vi "Init control.vi"(7 "ctl in":refnum<class "ctl.lvclass">, 8 "error in":errorcluster) -> (0 "error out":errorcluster, 3 "ctl out":refnum<class "ctl.lvclass">)   [LabVIEW 2012, in "ctl.lvclass"]
uses:
  ctl.lvclass
  Control Class/_ResourceManager_v86/ResManager/ID_Resource info.ctl
  ctl.lvclass/ctl.ctl
  Control Class/_ResourceManager_v86/ResManager/IDCloneResMgr.lvlib
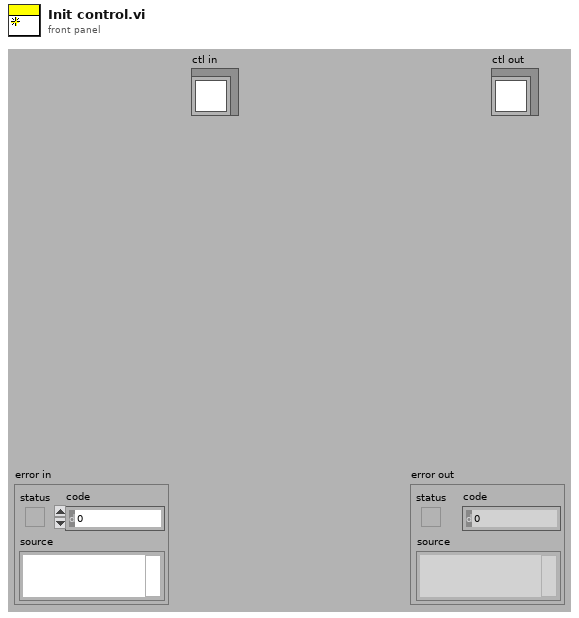
[diagram p1: front panel]
types:
  T1 = typedef "IDCloneResMgr.lvlib/ID_Resource info.ctl" = cluster{"type":u32, "id":i32, "name":string, "binary data":string}
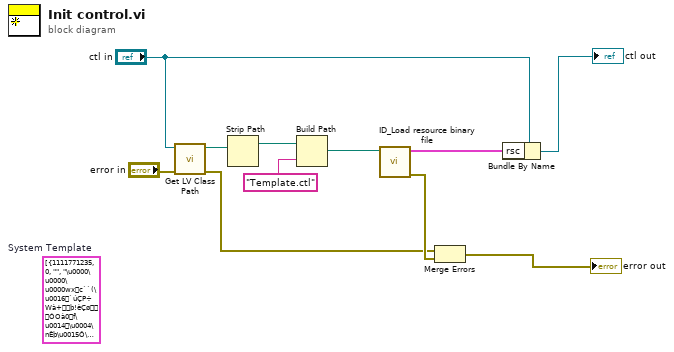
[diagram p0: block diagram]
diagram:
  (unwired) T1[] [{"type"=1111771235, "id"=0, "name"="", "binary data"="\u0000\u0000\u0000wxc``(\u0016`úÇP÷Wà+þ!èÇøÓOà0f\u0014\u0004\nÊþ\u0015Ô\u0006\u000bj³èª²1ªX1sHr\u001c\u0016ä\u0000q´h0üÿÿ_¥ã+Ë5\u0016\u001fYò\u001c\u0012\f\fÌ\f¸\f\u0000\u0004{\u0017´"}, {"type"=1111774021, "id"=0, "name"="", "binary data"="\u0000\u0000\u0000\u0007\u0000\u0000\u0001z"}, {"type"=1129270864, "id"=0, "name"="", "binary data"="\u0000\u0001"}, {"type"=1129333554, "id"=0, "name"="", "binary data"="\u0000\u0001"}, {"type"=1145455699, "id"=0, "name"="", "binary data"="\u0000\u0000\u0001\u0015xc`À\t\u0018\u0019\u0018X847Là?\u0010@Ä\u0005·Vò\u0001Ô\u000e\f6>1l@\u0000B1\u0002\u00153}\u00002\u0019À\u000e\u0007a¦?@ü\u000fY1#f\u0000Õ\u0001\u0014\u0018"}, {"type"=1146374224, "id"=0, "name"="", "binary data"="\u0000\u0002\u0000\u0010"}, {"type"=1179666531, "id"=0, "name"="", "binary data"="\u0000\u0000\u0004\u0006xS¿oÓ@\u0014~wuÜsià\\¨ \u0014ëÜ\u0004D°!è\u001a\u0017TT\n¨ø± \u00061T\u0004\u0012b\u0002©òâ¡,lþ\r\f\u0019X\u0011Ä\nY\u0015bghUK(6ïì\u0018÷G\u0010gÙïî½ï½ïî{g\u0000ò\u001c\rà¥ÏwÑ,õW{\u0004@©ð:ù\räTôYoÑ\u001402Ë.Ø.üÂè6FUÇ1ôOé7ÇÅûp3\u0018Ü \u0001½'{lÃic1pÊò«WH\u0000Ä>«(y»Ñj:Bzµ\nËGu4ßîe\n¯eäSZ\u0007°N\u0019:Î!älDxé?ÀgÂ;\u001f\u0001Ç\u0012 ]\fÞÈ­Iä!¼è!\u001c±/Rlÿêà\u0018Ft\fc}â\u000boåÙöê7½ã|\u0000\u0002Dy¨/KÕ\"ÀDßF%­ËÀWpu\u000bUR#]¥rT9r=RnÒv9¤'Ù\u0019.­tÍÑùv{­ÙhÅòq+&Ä82qÎ¡s\u001c·eýÕ5ë#³ö\\x\u0006²\b÷ÄA¹ÌPÀ\u001e®©Ö\u001a­GÍµó¨1O·Z\u0018@D[CSw÷ÈYiÔµ0\f\u0007Èc\u0012i\bo2¾jqL/Æ\u0017.N\u0019Ðxª¤ÓáÞÌ\u0001¯VÜß?ë>X\u000fÀöÇ¯ÈNb¯ØU\u001a\u00116nE[Þ'\u0013Ûâ\u000bóªo×&>f²Va/&z\u001dÅÄìE¶À7ñ7!>Ûd»ÊWeÉùB~Ðx[d9`xQª\u0000ä1½\t4òè0\r@çH\u001dt|q-çt\u000eýº\fËyø9tÉkÚép\u000f\nÃ*ë Û¢\"¦\n§á\u001aÚ\u00120\u0005ÇÁ\u0000#ü\u000e'1z\u0006ÖÃ\u0011Ç\f>MØÓñî\u000f&ñû\u000b"}, {"type"=1179669317, "id"=0, "name"="", "binary data"="\u0000\u0000\u0000\u0017\u0000\u0000\u0005N"}, {"type"=1179926850, "id"=128, "name"="", "binary data"="\u0000\u0001\u0000\u0002\u0000\u0003\u0000\u0005\u0000\u0000\u0000X\u0000\u000f\u0004\u0000\u0000\u0000\u0000\u000f\u0000Ø\u0000Õ\u0000\u0000\u0000a\u0000\u000f\u0004\u0000\u0000\u0000\u0000\u000f\u0000Ø\u0000Õ\u0000\u0000\u0000j\u0000\u000f\u0004\u0000\u0000\u0000\u0000\u000f\u0000Ø\u0000Õ\u0000\u0000\u0000s€\u0000„\u0000€\u0000\u0000\u000f\u0000Ø\u0000Õ\u0000\u0000\u0000u€\u0000„\u0000€\u0000\u0000\u000f\u0000Ø\u0000Õ\bSegoe UI\bSegoe UI\bSegoe UI\u00011\u00012"}, {"type"=1212765012, "id"=0, "name"="", "binary data"="\u0000\u0000\u0000\u0002\u0000\u0000\u0004\u0000\u0000\u0000\u0000\u000b\u0000\u0000\u0000\u0000\u0000\u0000\u0000\u0000\u0000\u0000\u0000\u0000\u0000\u0000\u0000\u0000\u0000\u0000\u0000\u0000\u0000\u0000\u0000\u0000\u0000\u0000\u0000\u0000"}, {"type"=1229147982, "id"=0, "name"="", "binary data"="ÿÿÿÿ\u0000\u0000\u0001\u0000\u0000\u0001@\u0000\u0001à\u0000\u0001ð\u0000\u0001\u0000\u0000\u0001à\u0000\u0001à\u0000\u0001à\u0000\u0001à\u0000\u0001ä\u0000\u0001ì\u0000\u0001Ô\u0000\u0001¤\u0000\u0001Ô\u0000\u0001ì\u0000\u0001ä\u0000\u0001à\u0000\u0001à0\u0001à,\u0001àã\u0001à$Áà.9à$Á\u0000ã\u0001ð,\u0001à0\u0001@\u0000\u0001\u0000\u0000\u0001\u0000\u0000\u0001ÿÿÿÿ"}, {"type"=1279877732, "id"=0, "name"="", "binary data"="\u0000\u0001BDHP\fTemplate.ctl\u0000\u0000\u0000\u0000\u0000\u0000\u0000\u0000\u0003"}, {"type"=1279878259, "id"=0, "name"="", "binary data"="\u0000\u0001VIDS\fTemplate.ctl\u0000\u0000\u0000\u0000\u0000\u0000\u0000\u0000\u0003"}, {"type"=1279878768, "id"=0, "name"="", "binary data"="\u0000\u0001FPHP\fTemplate.ctl\u0000\u0000\u0000\u0000\u0000\u0000\u0000\u0000\u0003"}, {"type"=1279882857, "id"=0, "name"="", "binary data"="\u0000\u0001LVCC\fTemplate.ctl\u0000\u0000\u0000\u0000\u0000\u0000\u0000\u0000\u0003"}, {"type"=1280725842, "id"=0, "name"="Template.ctl", "binary data"="\b`\u0001\u0000\u0000\u0000\u0000 \u0000\u0000\u0000\u0000\u0000\u0000\u0004\u0000\u0003\u0000<\u0000¼\u0000\u001f@\u0002\u0000\u0000\u0000\u0000\u0001\u0000\u0001\u0000\u0006ÿÿÿÿ\u0000\u0000\u0000\u0000\u0000\u0000\u0000\u0000\u0000\u0000\u0000\u0000m»+ånfN´ª¬¬\u001bcóz\u0000\u0000\u0000\f\u0000\u0000\u0000\u0010\u0000\u0000\u0000\u0002ñrÈFô}vG§qnâÃ¸Ô\u001dÙ\u0000²\u0004é\tìøB~\u0000\u0000@\u0000\u0000\u0000\u0000\u0000"}, {"type"=1296975689, "id"=2, "name"="", "binary data"="PNG\r\n\u001a\n\u0000\u0000\u0000\rIHDR\u0000\u0000\u0000\u0016\u0000\u0000\u0000\u0016\b\u0006\u0000\u0000\u0000Ä´l;\u0000\u0000\u0000\u0004gAMA\u0000\u0000¯È7\u0005é\u0000\u0000\u0000\u0019tEXtSoftware\u0000Adobe ImageReadyqÉe<\u0000\u0000\u0004:IDATxÚbüÿÿ?\u0003-\u0000@\u000011Ð\b\u0000\u0004 pÜ\u0000\u0004(¸|N\f´\u00023Û±\b±\u0010t\u0019àÀ#y»Á\u0006/ÎÙù<v!\u0015i1Ñ\u00154V4\u00144ª+ ÊHæL7úÊ°\u0006¯×²¥×{÷å;¿\u0000¢ØÅà üó·EJLt]¨µ¨\u0010<H\u001c X(1ôÏ\fl\fëLuÔÌãÍõ\u00197]½ÇðêÉÇÍ 9\u0000\"ËÅ@üûÏ_\u0006\u000eÖóA6\u0006\u0016]nögî¿dØuäæ¥¿ÿÔ\u0000\u0004\u0010\u000bÔ;\u0002ÿÿýg\u00032_\u0011ôú¿ÿ\fß~ýí\u0013\u0015ÈIrÐd\rWVbXxõ.ÃâÝ×\u001e3þftcd\u0005E\u0004\u0003\u0003@\u0000\ræàd?öAôÏû¿^Ì\f\f§q\u0019ú÷ïÉ_,ÿ×iéHXä;ê08\b\u000b3Ì¹yaúæ«\u001f\u0018¿ýscæfxùñ\u001fX-@\u0000[ÅÖZNmÛß?ÿÁ~E\u0003¿ÿ\u000b`âe>ïf§hÑìiÍ`%,É°êÁcÙ[îü`üÀ\u0018ÉÆÌvå/\u001b\u0003Ëo\u000e°z\u0000\u0002\u001büþé3\n\\Ü\fÁnª\"Xÿ\u001føûç¿,Âë\f\f¿þüÉ+Ã¶:ÅOW¼ÜÖASaë£G\fÓ×Ýÿûëù¿$nv¶\u001dìÿ¸\u0019¸~\n0ð|\u0011\u0001ë\u0003\b °Áÿ¿2M>qæýÿ0\u001d\u000b\u0006\u001fG5\u001f÷üûÃÀ\u0001²à'óß\u0013*\u0006..."}, {"type"=1296975689, "id"=3, "name"="", "binary data"="PNG\r\n\u001a\n\u0000\u0000\u0000\rIHDR\u0000\u0000\u0000\u0000\u0000\u0000\u001e\b\u0006\u0000\u0000\u0000à§ÆÅ\u0000\u0000\u0000\u0001sRGB\u0000®Î\u001cé\u0000\u0000\u0000\u0004gAMA\u0000\u0000±\u000büa\u0005\u0000\u0000\u0000\tpHYs\u0000\u0000\u000eÃ\u0000\u0000\u000eÃ\u0001Ço¨d\u0000\u0000\u0000\u0019tEXtSoftware\u0000Paint.NET v3.5.1Nç8ù\u0000\u0000\u0001LIDAThCíA.DA\u0014EÿÈ\u0012\fÌíÂ\u0016L{#¬Â\u001aÌåK\u0004ÐBBÆ\u001f MH´DcÐ§êu{I%vpO%7\\§Î»õ'Õ4óµÜÛ´fe\b1X\\Ýxÿ;ÿÙ7o~ïìÎXZ\u0004.»ç2ø[y×ÛMnµ¶«EÝ\u0006¶?4¿\rJ\u001b¤(bÿ\u0012 ö\u0010 h\u0003ü×þÑ\b?ÓdDAð9IöõMT\u0019T\"\u0014\u0019&\u0003D@~\u001f~D@ZñÇÔ.h\u0004$Ð =\"Ð~\u0013\b/¯\u0013#º\f\u0010\u0001ð\u0002\b\u0011\u001eÆFt\u0019 \u0002\u0003à\u0005\bPpß½\u0019Ñe\u0010\u0004º\u0012³G\u0004Ðo\u0010áúfdD\u0001\"0\u0000^\u0000\bW\u0011=\u0006\b\u0017çFt\u0019D#tFt\u0019¸\bùÙµGÇvx0 ¢\f\u0003ñämgw\u001f\u0011\u0004E]\u000bó\u001f9,ð\bVï\u0001pi¼\u0006¿ÊÊÚí¥Ö\u0000\u0000\u0000\u0000IEND®B`"}, {"type"=1296975689, "id"=4, "name"="", "binary data"="PNG\r\n\u001a\n\u0000\u0000\u0000\rIHDR\u0000\u0000\u0000\u0000\u0000\u0000\u001e\b\u0006\u0000\u0000\u0000à§ÆÅ\u0000\u0000\u0000\u0001sRGB\u0000®Î\u001cé\u0000\u0000\u0000\u0004gAMA\u0000\u0000±\u000büa\u0005\u0000\u0000\u0000\tpHYs\u0000\u0000\u000eÃ\u0000\u0000\u000eÃ\u0001Ço¨d\u0000\u0000\u0000\u0019tEXtSoftware\u0000Paint.NET v3.5.1Nç8ù\u0000\u0000\u0001yIDAThCí1N\u0002Q\u0010W\u000fá\r¸\u0017°°õ\u001c\u0016ÔVÀÞR\u0003\r\u0018³\u0016lÄd7D\b\u00180Á\u0004*M°m\u0004Â\u000eoî-µäÿ7ùYÚ÷Í7ó( øyJG§\u0012ì\u0019 \u0006{'i^ÿ>8>óðÁ\"P\u000fCÑÚ{\tÜ$\u0018Tªu©U#\u0006Áåu$Îç@¯«FÂ\u00003ð?\tôã&ì0À\fLfÔ\u0013\u0006pÛê\tË\"°\u0001ü\u00000\u0011âd(\f.\u0003°\rÐûnj°\"üg²\b÷Ý0¸\f(\u0002\u001bÀ\u000f\u0000@\u0011\"<\f&Âà2°@\tp%ÐÚ\b£§\u0017ap\u0019P\u00046\u001f\u0000\u0014\"\u0014E\u0018O¦Âà2°@\tp%ÐÚS\u0004NB\u0013\bÓ×T\u0018\\\u0006&ÂÛl.yféB\u0018,\u0006&Âûb%yæËµ08\fô\u000fü&\u0016~ùéòµ\u0015Ä  Be\u0007kÅ§5\u0011ÜÚ46\u0012ûÃïm'wþ\u001dýÒ¸ë¢À=vçqü»ò¦ko\u000eÅ.`ñ\u0016õ6ÐA \u000el\u0000>¸¬pýùàÕ\u0000\u0000\u0000\u0000IEND®B`"}, {"type"=1296975689, "id"=5, "name"="", "binary data"="PNG\r\n\u001a\n\u0000\u0000\u0000\rIHDR\u0000\u0000\u0000\u0000\u0000\u0000\u001e\b\u0006\u0000\u0000\u0000à§ÆÅ\u0000\u0000\u0000\u0001sRGB\u0000®Î\u001cé\u0000\u0000\u0000\u0004gAMA\u0000\u0000±\u000büa\u0005\u0000\u0000\u0000\tpHYs\u0000\u0000\u000eÃ\u0000\u0000\u000eÃ\u0001Ço¨d\u0000\u0000\u0000\u0019tEXtSoftware\u0000Paint.NET v3.5.1Nç8ù\u0000\u0000\u0002$IDAThCí=KÃ`\u0014ó+ü\u0007Îº¸¨.ÚAÐEtÓÁAA¤ÅA+\bÚ*(K¥  ¢KµT\n\u0015EAé`±â÷'Tñ£\u0015¬&iâõ½\tM\u0002NÃ½CÚ¥s{îKá$ñ\u001a\b-\u0007Ê[ Õö³\byPÖ4\f¡\u0015@\u0006\u0010ÞéEÈ>¥\u0001r)\u0016!\u000fä·cÀì\r\u0018°\tÞ¯×@K\u000f~>Á\"ä\u0001fÙ\u001bÛ\u0000×ÁÏÝ\t®³\by`d~?o\u001e\u0007\f\u0010nf\u0019\u0004B\u0000\u0014\u0007\u001eAÀì-\u0010ô«\u0019\u0006(\b½\rØ¼\u001aè­Åâ¹Ð\u0006ádA Ú\b'#v#hi¿\u0000Á\u000f²¦³\by \u001dù\u0019\u0004êà3\b¦¾\u0014ìn\u0010\u000e½ \t}}ë,B\u001e\u0014R>»Ï±\u001a\u0018\u0004\u0003À \u0010úR-ï\u0006!Ù\rd\u000f|æu\u0016!\u000f0sMdoý\u001f\u0018\u0004zCà\u0002¡°ß\t\u000eÈ}h,B\u001e¨»Õ\b\f\u0002Í\u0001`\u0010\bM}©w î¶º×\u000eÏ/y\u0016!\u000fÔ=3wk50\b4\u0007A 4õ¥ZÞ\rÂv3¨;Íððc\u0011ò@Ýn1r·VðºåÛ»W\u0016!\u000fT»ht\u0011âu Äëáâ2Ã\"äbä^çhÍ\u001aPb5\f\u0001!\bpèe¹\u0012«v°Q\u0005r´\nNÏ2,B\u001e`æ²ÈÞ8#àµ§..."}, {"type"=1297434948, "id"=0, "name"="", "binary data"="\u0000\u0000\u0000P"}, {"type"=1381258055, "id"=0, "name"="", "binary data"="\u0000\u0000\u0000\u0000\u0000\u0000\u0000\u0000\u0000\u0000\u0000\u0000\u0000\u0000\u0000\u0000"}, {"type"=1414346800, "id"=0, "name"="", "binary data"="\u0000\u000e\u0000\u0002\u0010\u0000\u0010\u0001\u0010\u0000\u0010\u0004\u0010\u0000\u0010\u0000\u0010\u00000\u0000\u0010\u0000\u0010\u0000\u0010\u00000\u0000\u0010\b\u0010\u0000"}, {"type"=1447253072, "id"=0, "name"="", "binary data"="\u0000\u0000\u0001exU½nÂ@\u0010?û\u0000CðO\u0002!\u0005=\r\u00125²P\u001e\u0000å\t@Ø¦±r(hò°y\fw(\u001aévgwng\u0017x§\u0015Ï£µyºÿâ\u0003\u0004?T¨b\u0010M%!uvÊZªlÅ\u0004NÊF\u001ca²üH=¾\u0018ûYøBj3ºñVÚH¿\u001bæd\u0012ÌM%.\u0016g\u001fmîcz.èkzM¡)¯6Ï¥ËB.>3Êj\\¹ï\u0016\n¾óñÐ|?¶Ã\u001d\u0012¢' ¼¡ÂZ.3^×\u0012¡ÃöÇï8xß©&AÏåUíÔ¡+ÖgÀ\u0011cÞÔÝVø\u0005³g\u001e\u000b"}, {"type"=1447641924, "id"=0, "name"="", "binary data"="\u0000\u0000\u0001\u0004xëa``È4¶0;Á\u0000Éù)© ú\u0003\u0010w¾Øg\b¢\nx;è\b\u0002Y\u0001¡Ý®\fÿ\u0005zST8lAJÙw¨Ã\u0013þ?0aB|\\Tdtìá\t¡Ý9*\u001cÁAaáÝ%**Ý5*\u001aüûØø÷É[ÜØÁ\bT]Â\nÖTÊ\næaÑTÊ°#\u001cd­Æ\u000e\u00050í°£\u0007L»dt¾\u0000i\u0007¹\u0001¦\u0017dÞa \u0014Hö?\u0010ä\u0019\u0019X\u0018\u0019f1,bX\u0005÷³¿+WÁ~\u0004\u0000·ý@M"}, {"type"=1768123448, "id"=0, "name"="", "binary data"="ýýýýýýýýýýýýýýýýýýýýýýýýýýýýýýýýý\u0000\u0000\u0000\u0000\u0000\u0000\u0000\u0000\u0000\u0000\u0000\u0000\u0000\u0000\u0000\u0000\u0000\u0000\u0000\u0000\u0000\u0000\u0000\u0000\u0000\u0000\u0000\u0000\u0000\u0000ýý\u0000\u0000\u0000\u0000\u0000\u0000\u0000\u0000\u0000\u0000\u0000\u0000\u0000\u0000\u0000\u0000\u0000\u0000\u0000\u0000\u0000\u0000\u0000\u0000\u0000\u0000\u0000\u0000\u0000\u0000ýý\u0000\u0000\u0000\u0000\u0000\u0000\u0000\u0000+\u0000\u0000\u0000\u0000\u0000\u0000\u0000\u0000\u0000\u0000\u0000\u0000\u0000\u0000\u0000\u0000\u0000\u0000\u0000\u0000\u0000ýý\u0000\u0000\u0000\u0000\u0000\u0000\u0000+¬\u0000\u0000\u0000\u0000\u0000\u0000\u0000\u0000\u0000\u0000\u0000\u0000\u0000\u0000\u0000\u0000\u0000\u0000\u0000\u0000ýý\u0000\u0000\u0000\u0000\u0000\u0000+úùúù\u0000\u0000\u0000\u0000\u0000\u0000\u0000\u0000\u0000\u0000\u0000\u0000\u0000\u0000\u0000\u0000\u0000\u0000\u0000ýý\u0000\u0000\u0000ùùV\u0000\u0000\u0000\u0000\u0000\u0000\u0000\u0000\u0000\u0000\u0000\u0000\u0000\u0000\u0000\u0000\u0000\u0000\u0000\u0000\u0000\u0000\u0000\u0000ýý\u0000\u0000\u0000\u0000\u0000\u0000\u0000àþý\u0000\u0000\u0000\u0000\u0000\u0000\u0000\u0000\u0000\u0000\u0000\u0000\u0000\u0000\u0000\u0000\u0000\u0000\u0000\u0000ýý\u0000\u0000\u0000\u0000\u0000\u0000\u0000þüý\u0000\u0000\u0000\u0000\u0000\u0000\u0000\u0000\u0000\u0000\u0000\u0000\u0000\u0000\u0000\u0000\u0000\u0000\u0000\u0000ýý\u0000\u0000\u0000\u0000\u0000\u0000\u0000¬üý\u0000\u0000\u0000\u0000\u0000\u0000\u0000\u0000\u0000\u0000\u0000\u0000\u0000\u0000\u0000\u0000\u0000\u0000\u0000\u0000ýý\u0000\u0000\u0000\u0000\u0000\u0000\u0000þüà\u0000\u0000\u0000\u0000\u0000\u0000\u0000\u0000\u0000\u0000\u0000\u0000\u0000\u0000\u0000\u0000\u0000\u0000\u0000\u0000ýý\u0000\u0000\u0000\u0000\u0000\u0000\u0000þ¬ý\u0000øú\u0000\u0000\u0000\u0000\u0000\u0000\u0000\u0000\u0000\u0000\u0000\u0000\u0000\u0000\u0000\u0000\u0000ýý\u0000\u0000\u0000ùùV\u0000þ¬¬Vu¦\u0000\u0000\u0000\u0000\u0000\u0000\u0000\u0000\u0000\u0000\u0000\u0000\u0000\u0000\u0000\u0000\u0000ýý\u0000\u0000\u0000\u0000\u0000\u0000+P&Ju¬+\u0000\u0000\u0000\u0000\u0000\u0000\u0000\u0000\u0000\u0000\u0000\u0000\u0000\u0000\u0000\u0000ýý\u0000\u0000\u0000\u0000\u0000VüJutu¬+\u0000\u0000\u0000\u0000\u0000\u0000\u0000\u0000\u0000\u0000\u0000\u0000\u0000\u0000\u0000\u0000ýý\u0000\u0000\u0000\u0000\u0000\u0000öþ¬¦uv¬+\u0000\u0000\u0000\u0000\u0000\u0000\u0000\u0000\u0000\u0000\u0000\u0000\u0000\u0000\u0000\u0000ýý\u0000\u0000\u0000\u0000\u0000\u0000õàþþüÊ¬+\u0000\u0000\u0000\u0000\u0000\u0000\u0000\u0000\u0000\u0000\u0000\u0000\u0000\u0000\u0000\u0000ýý\u0000\u0000\u0000\u0000\u0000\u0000\u0000¬¬þõVû+\u0000\u0000\u0000\u0000\u0000\u0000\u0000\u0000\u0000\u0000\u0000\u0000\u0000\u0000\u0000\u0000ýý\u0000\u0000\u0000ùùV\u0000þûà\u0000\u0000++\u0000\u0000\u0000\u0000\u0000\u0000\u0000\u0000\u0000..."}, {"type"=1986359923, "id"=4, "name"="", "binary data"="\b`€\u0001\u0000\u0000\u00038.6\u0000"}]  # System Template
  n1 = call <vilib>:"Get LV Class Path.vi"("error in (no error)"="error in", "object"="ctl in") -> ("error out"=w3:errorcluster, "class path"=w7:path)  [unwired: 8 out]
  n2 = Strip Path(path=w7) -> (stripped path=w2:path)  [unwired: 1 out]
  n3 = Build Path(base path=w2, name or relative path="Template.ctl") -> (appended path=w5:path)
  n4 = call "ID_Load resource binary file.vi"("resource binary file"=w5) -> ("error out"=w10:errorcluster, "resources"=w1:T1[])  [unwired: 9 out]
  n5 = Merge Errors(w3, w10) -> (→"error out":errorcluster)
  n6 = Bundle By Name(cluster="ctl in", "rsc"=w1) -> (→"ctl out":refnum<class "ctl.lvclass">)
